vi "Tree结合嵌套Tab.vi"() -> ()   [LabVIEW 2013]
panel:
  out "DAQ":enum32{"DAQ01", "DAQ02"}(tab)
  out "DAQ01":T1(tab)
  out "DAQ02":T2(tab)
  in  "Stop":bool
  in  "Select Page Tree":string(tree)
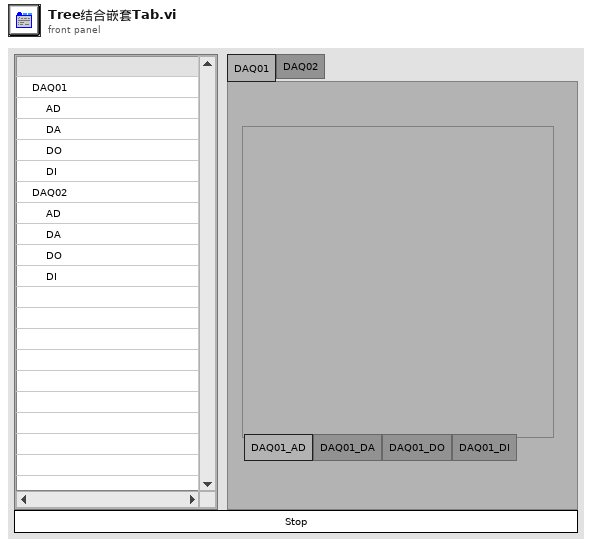
[diagram p1: front panel]
types:
  T1 = enum32{"DAQ01_AD", "DAQ01_DA", "DAQ01_DO", "DAQ01_DI"}
  T2 = enum32{"DAQ02_AD", "DAQ02_DA", "DAQ02_DO", "DAQ02_DI"}
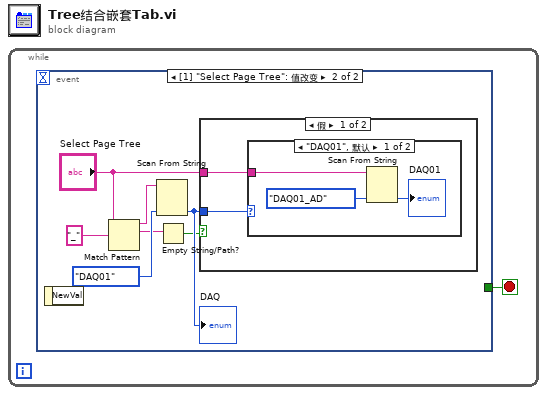
[diagram p0: block diagram]
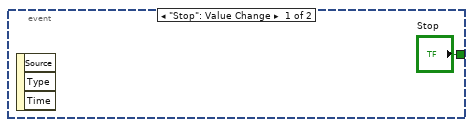
[diagram p2: hidden frame]
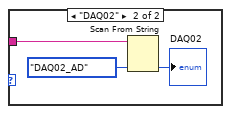
[diagram p3: hidden frame]
diagram:
  n1 = while {
    stop <- w1 stop-if-true
    n2 = event shown="[1] \"Select Page Tree\": 值改变" {
      selector: _ -> [_ _]
      dyn-events: _ -> [_ _]
      timeout: _ -> [_ _]
      tunnel: ["Stop" _] -> w1
      event "Stop": Value Change {
        n3 = event-data() -> ()  [unwired: 1 in, 3 out]
      }
      event "Select Page Tree": Value Change {
        n4 = event-data() -> ()  [unwired: 1 in, 1 out]
        n5 = Match Pattern(string="Select Page Tree", regular expression="_" ("替换字符串(\"\")")) -> (before substring=w7:string, match substring=w4:string)  [unwired: 1 in, 2 out]
        n6 = Scan From String(input string=w7, default 1=enum32{"DAQ01", "DAQ02"}."DAQ01" ("DAQ")) -> (output 1=w5:enum32{"DAQ01", "DAQ02"})  [unwired: 3 in, 3 out]
        "DAQ" <- w5
        n7 = Empty String/Path?(string/path=w4) -> (empty?=w3:bool)
        n8 = case shown="假" w3 {
          tunnel: w5 -> [w11 _]
          tunnel: "Select Page Tree" -> [w10 _]
          frame False {
            n9 = case shown="\"DAQ01\", 默认" w11 {
              tunnel: w10 -> [w14 w16]
              frame "DAQ01", Default {
                n10 = Scan From String(input string=w14, default 1=T1."DAQ01_AD" ("DAQ01")) -> (output 1=→"DAQ01":T1)  [unwired: 3 in, 3 out]
              }
              frame "DAQ02" {
                n11 = Scan From String(input string=w16, default 1=T2."DAQ02_AD" ("DAQ02")) -> (output 1=→"DAQ02":T2)  [unwired: 3 in, 3 out]
              }
            }
          }
          frame True {
          }
        }
      }
    }
  }
